vi "CreatePublicEvents.vi"(8 "error in (no error)":errorcluster, 11 "DSP":refnum<class "DSP.lvclass">) -> (0 "error out":errorcluster, 3 "DSP out":refnum<class "DSP.lvclass">)   [LabVIEW 2016, in "DSP.lvclass"]
doc: "---------------------------------------------------------------\nJKI State Machine Objects™\nhttp://jki.net/state-machine-objects/\nCopyright (C) 2005-2015, JKI <info@jki.net>\nALL RIGHTS RESERVEDJKI State Machine Objects (SMO) 1.0.0.4\nJKI - JKI\nCopyright (c) 2015, JKI"
uses:
  DSP.lvclass
  Typedefs/PublicEvents--DSP.getWaveforms.ctl
  Typedefs/PublicEvents--DSP.getLockin.ctl
  DSP.lockin/Typedefs/LockinResult.ctl
  Typedefs/PublicEvents--DSP.getPowerSpectrum.ctl
  DSP.lvclass/DSP.ctl
  <vilib>/JKI/JKI SMO/SMO/SMO.lvclass
  DSP.lockin/DSP_lockin.lvclass
panel:
  # "For instructions on how to use the JKI State Machine Objects, examples and video tutorials, visit:\nhttp://jki.net/state-machine-objects/\n\nJKI State Machine Objects™\nhttp://jki.net/state-machine-objects/\nCopyright (C) 2005-2015, JKI <info@jki.net>\nALL RIGHTS RESERVED"
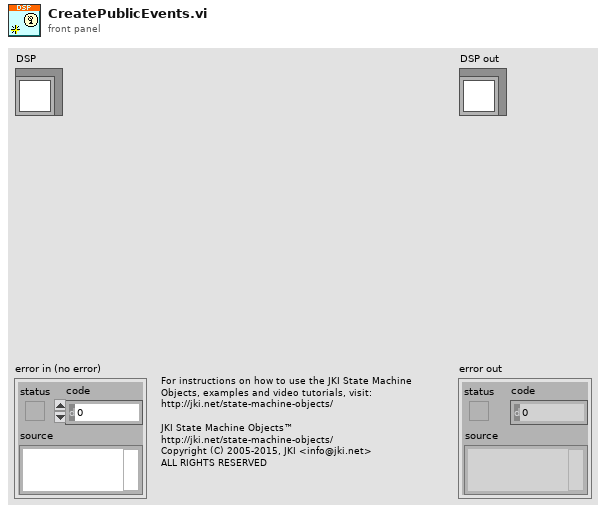
[diagram p1: front panel]
types:
  T1 = typedef "DSP.lvclass/PublicEvents--DSP.getPowerSpectrum.ctl" = cluster{"f0":dbl, "df":dbl, "magnitude":dbl[]}[]
  T2 = typedef "DSP.lvclass/PublicEvents--DSP.getLockin.ctl" = T3[]
  T3 = typedef "DSP_lockin.lvclass/LockinResult.ctl" = cluster{"X":dbl, "Y":dbl, "R":dbl, "Theta":dbl, "AVG":dbl, "f":dbl}
  T4 = typedef "PublicEvents--DSP.getWaveforms.ctl" = waveform(dbl)[]
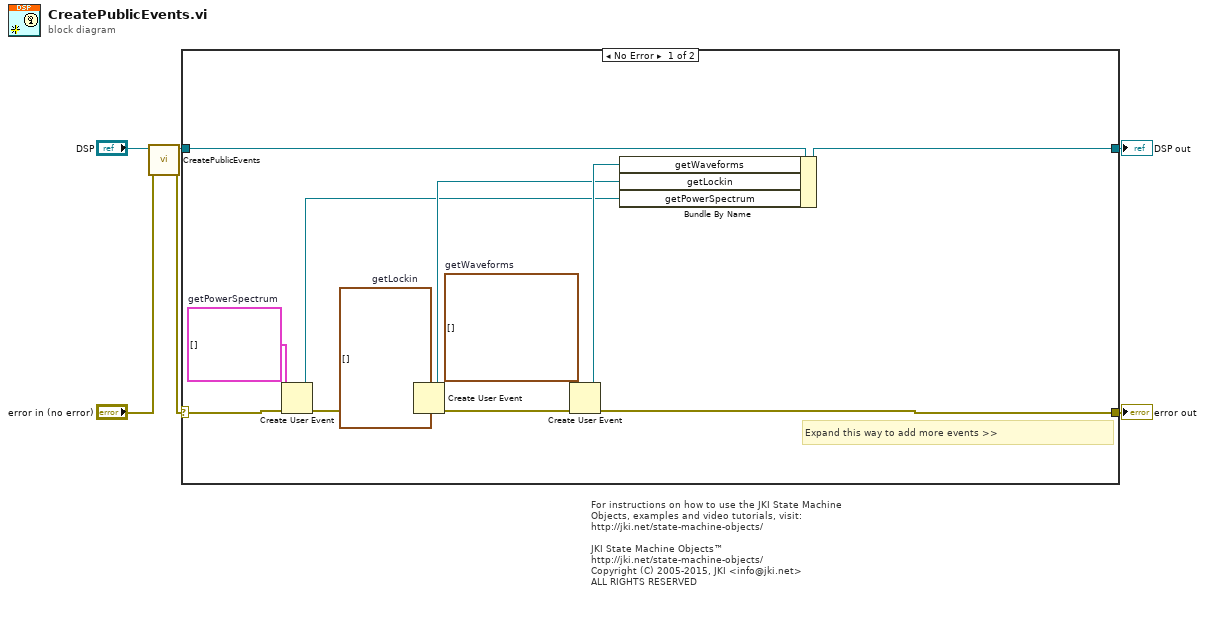
[diagram p0: block diagram]
diagram:
  # "For instructions on how to use the JKI State Machine Objects, examples and video tutorials, visit:\nhttp://jki.net/state-machine-objects/\n\nJKI State Machine Objects™\nhttp://jki.net/state-machine-objects/\nCopyright (C) 2005-2015, JKI <info@jki.net>\nALL RIGHTS RESERVED"
  n1 = call-parent "CreatePublicEvents.vi"("error in (no error)"="error in (no error)", "SMO"="DSP") -> ("error out"=w1:errorcluster, "SMO out"=w3:refnum<class "DSP.lvclass">)  [unwired: 8 in]
  n2 = case shown="No Error" w1 {
    selector: w1 -> [w17 w20]
    tunnel: [w15 w20] -> w5
    tunnel: [w16 w19] -> w6
    tunnel: w3 -> [w18 w19]
    frame No Error {
      w8 = T1 []  # getPowerSpectrum
      w11 = T2 []  # getLockin
      w14 = T4 []  # getWaveforms
      # "Expand this way to add more events >>"
      n3 = Create User Event(user event datatype=w8, error in=w17) -> (user event=w7:refnum<user-event>, error out=w9:errorcluster)
      n4 = Create User Event(user event datatype=w11, error in=w9) -> (user event=w10:refnum<user-event>, error out=w12:errorcluster)
      n5 = Create User Event(user event datatype=w14, error in=w12) -> (user event=w13:refnum<user-event>, error out=w15:errorcluster)
      n6 = Bundle By Name(cluster=w18, "getWaveforms"=w13, "getLockin"=w10, "getPowerSpectrum"=w7) -> (w16:refnum<class "DSP.lvclass">)
    }
    frame Error {
    }
  }
  "error out" <- w5
  "DSP out" <- w6
